vi "frequency_counter.vi"() -> ()   [LabVIEW 2012]
panel:
  in  "InputB CH1":dbl[](array[numeric])
  in  "Input A CH0":dbl[](array[numeric])
  out "error out":errorcluster
  in  "error in (no error)":errorcluster
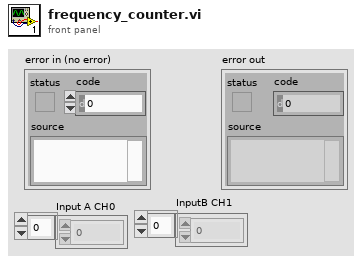
[diagram p1: front panel]
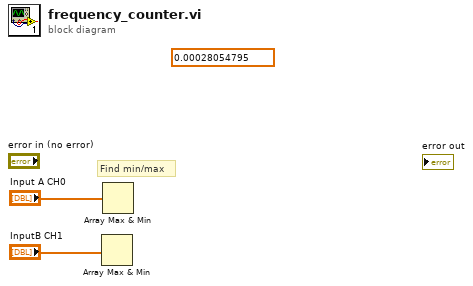
[diagram p0: block diagram]
diagram:
  (unwired) 0.00028054795 ("dt")
  # "Find min/max"
  n1 = Array Max & Min(array="InputB CH1") -> ()  [unwired: 4 out]
  n2 = Array Max & Min(array="Input A CH0") -> ()  [unwired: 4 out]
